vi "RT_Control_Adrian_ESP.vi"(10 "rt fifo":refnum<k33>, 11 "Parameters":T1={"N_chan"=0, "Input Rate (Hz)"=0.0, "Acq Time (s)"=0.0, "NumOfWarmupIters"=0, "Size fifo"=0, "Period NCL (ms)"=0, "Timeout fifo Read"=0, "Size Sent Array"=0, "Output offsets"=[], "Input offsets"=[0.0, 0.0, 0.0, 0.0, 0.0, 0.0, 0.0, 0.0]}) -> (0 "error out":errorcluster, 2 "Delayed Cycles":dbl)   [LabVIEW 2021]
uses:
  parametersRT.ctl
  <vilib>/DAQmx/write.llb/DAQmx Write (Analog 1D DBL NChan 1Samp).vi
  <vilib>/DAQmx/read.llb/DAQmx Read (Analog 1D DBL NChan 1Samp).vi
  <vilib>/DAQmx/write.llb/DAQmx Write (Digital Bool 1Line 1Point).vi
  <vilib>/DAQmx/create/channels.llb/DAQmx Create Channel (DO-Digital Output).vi
  <vilib>/DAQmx/configure/timing.llb/DAQmx Timing (Sample Clock).vi
  <vilib>/DAQmx/miscellaneous.llb/DAQmx Fill In Error Info.vi
  <resource>/objmgr/daqmx.rc
panel:
  out "timed out?":bool
  out "# elements":u32
  out "data":dbl[](array[numeric]) format="%0.2f"
  out "Numeric":i32
  out "output array":dbl[](array[numeric])
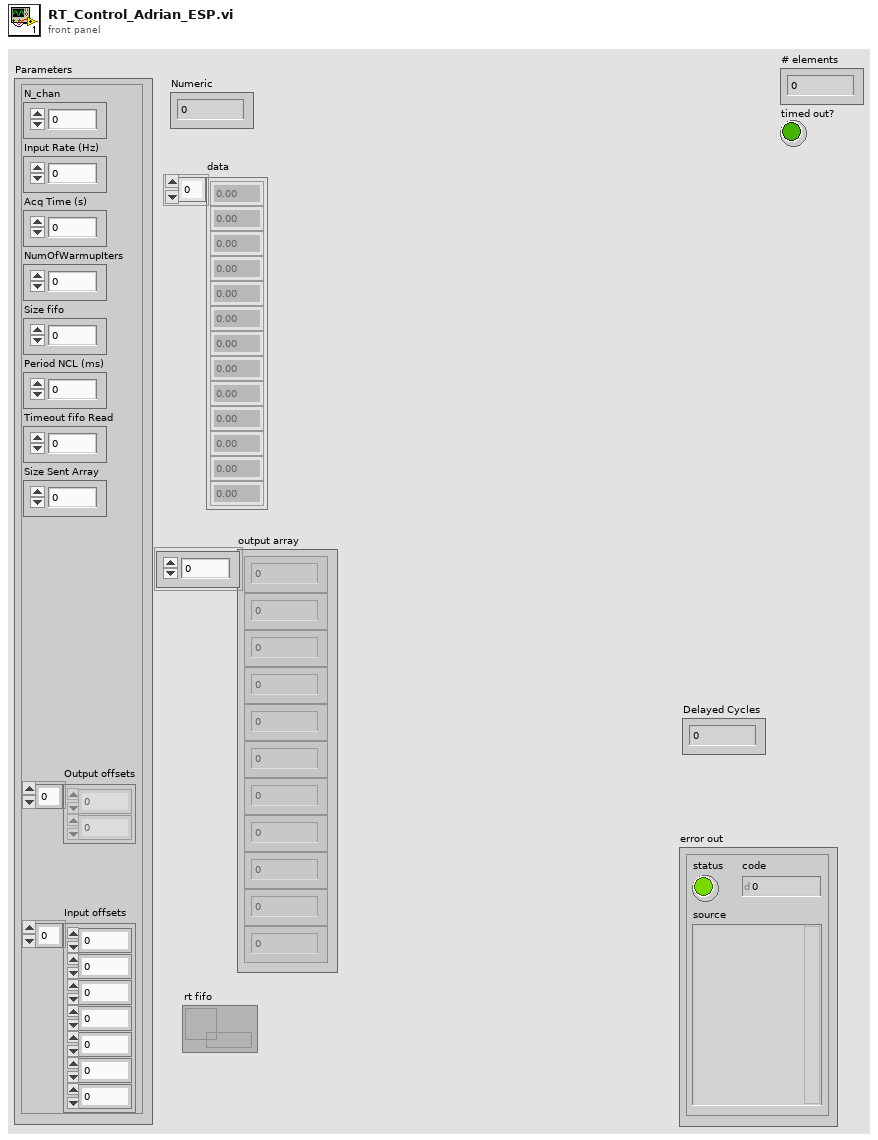
[diagram p1: front panel]
types:
  T1 = typedef "parametersRT.ctl" = cluster{"N_chan":u32, "Input Rate (Hz)":dbl, "Acq Time (s)":dbl, "NumOfWarmupIters":u32, "Size fifo":u32, "Period NCL (ms)":i64, "Timeout fifo Read":i32, "Size Sent Array":i32, "Output offsets":dbl[], "Input offsets":dbl[]}
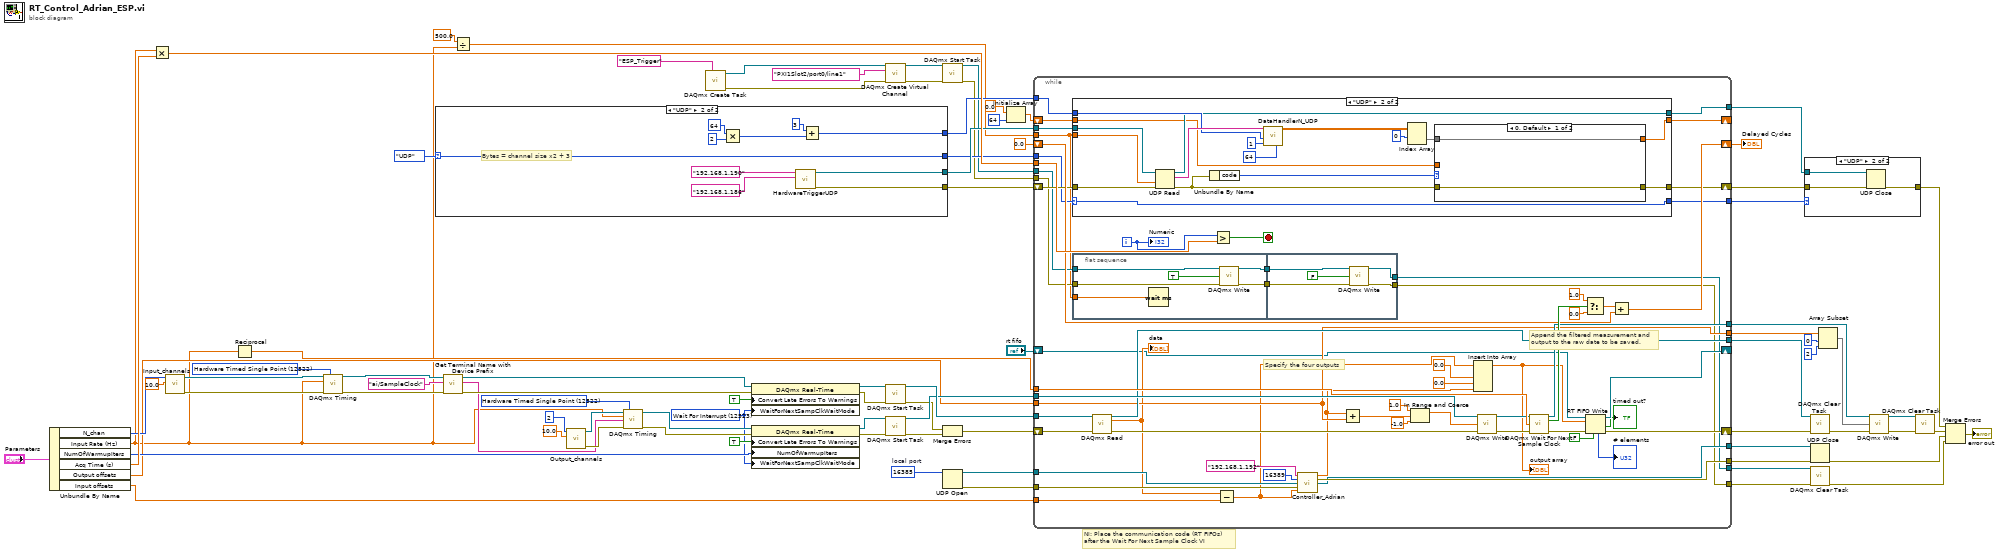
[diagram p0: block diagram]
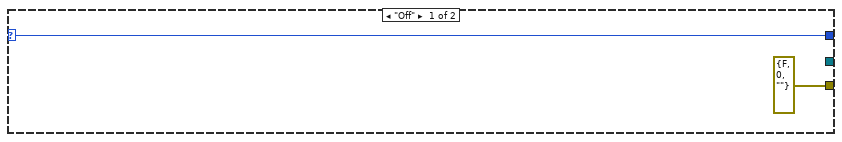
[diagram p3: hidden frame]
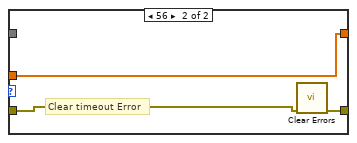
[diagram p5: hidden frame]
diagram:
  w42 = u16 16385  # local port
  w49 = 12522 items=["Finite Samples"=10178, "Continuous Samples"=10123, "Hardware Timed Single Point"=12522] ("sample mode")
  w57 = 12523 items=["Wait For Interrupt"=12523, "Poll"=12524, "Yield"=12525] ("WaitForNextSampClkWaitMode")
  w83 = 12522 items=["Finite Samples"=10178, "Continuous Samples"=10123, "Hardware Timed Single Point"=12522] ("sample mode")
  # "NI: Place the communication code (RT FIFOs) \nafter the Wait For Next Sample Clock VI"
  n1 = Unbundle By Name("Parameters") -> ("N_chan"=w68:u32, "Input Rate (Hz)"=w17:dbl, "NumOfWarmupIters"=w69:u32, "Acq Time (s)"=w76:dbl, "Output offsets"=w67:dbl[], "Input offsets"=w58:dbl[])
  n2 = Multiply(x=w17, y=w76) -> (x*y=w36:dbl)
  n3 = call "Input_channels.vi"("Range"=10.0, "nchan"=w68) -> ("error out"=w51:errorcluster, "Refnum out"=w50:refnum<k21>)  [unwired: 8 in]
  n4 = Reciprocal(x=w17) -> (1/x=w82:dbl)
  n5 = call-poly <vilib>:"DAQmx Timing.vi"("task/channels in"=w50, "sample mode"=w49, "rate"=w17, "error in"=w51) -> ("task out"=w30:refnum<k21>, "error out"=w32:errorcluster)  [unwired: 10 in]
  n6 = case shown="\"UDP\"" enum16{"Off", "UDP"}."UDP" {
    selector: enum16{"Off", "UDP"}."UDP" -> [w86 w89]
    tunnel: [_ w92] -> w23
    tunnel: [errorcluster {"status"=FALSE, "code"=0, "source"=""} ("error constant") w90] -> w25
    tunnel: [w86 w89] -> w22
    tunnel: [_ w88] -> w24
    frame "Off" {
    }
    frame "UDP" {
      # "Bytes = channel size x2 + 3"
      n7 = Multiply(x=64, y=2) -> (x*y=w95:i32)
      n8 = call "HardwareTriggerUDP.vi"("Local IP address"="192.168.1.186" ("Hardware Trigger"), "Remote IP address"="192.168.1.190" ("IP address")) -> ("error out"=w90:errorcluster, "connection ID out"=w88:refnum<k16>)  [unwired: 8 in]
      n9 = Add(x=3, y=w95) -> (x+y=w92:i32)
    }
  }
  n10 = call "Get Terminal Name with Device Prefix.vi"("error in (no error)"=w32, "Local Terminal Name"="ai/SampleClock", "task/channels in"=w30) -> ("error out"=w31:errorcluster, "Terminal Name with Device Prefix"=w28:tag, "task out"=w29:refnum<k21>)  [unwired: 6 in]
  n11 = Divide(x=500.0, y=w17) -> (x/y=w16:dbl)
  n12 = call "Output_channels.vi"("Range"=10.0 ("Maximum Value"), "nchan"=2) -> ("error out"=w73:errorcluster, "Refnum out"=w72:refnum<k21>)  [unwired: 8 in]
  n13 = call-poly <vilib>:"DAQmx Timing.vi"("task/channels in"=w72, "sample mode"=w83, "rate"=w17, "source"=w28, "error in"=w73) -> ("task out"=w81:refnum<k21>, "error out"=w80:errorcluster)  [unwired: 9 in]
  n14 = call <vilib>:"DAQmx Create Task.vi"("new task name"="ESP_Trigger") -> ("task out"=w13:refnum<k21>, "error out"=w12:errorcluster)  [unwired: 13 in]
  n15 = property class="DAQmx Real-Time"(reference=w29, error in=w31, "Convert Late Errors To Warnings"=TRUE, "WaitForNextSampClkWaitMode"=w57) -> (reference out=w46:refnum<k21>, error out=w45:errorcluster)
  n16 = property class="DAQmx Real-Time"(reference=w81, error in=w80, "Convert Late Errors To Warnings"=TRUE, "NumOfWarmupIters"=w69, "WaitForNextSampClkWaitMode"=w57) -> (reference out=w77:refnum<k21>, error out=w54:errorcluster)
  n17 = call-poly <vilib>:"DAQmx Create Virtual Channel.vi"("task in"=w13, "lines"=tag "PXI1Slot2/port0/line1", "error in"=w12) -> ("task out"=w11:refnum<k21>, "error out"=w10:errorcluster)  [unwired: 11 in]
  n18 = call <vilib>:"DAQmx Start Task.vi"("task/channels in"=w46, "error in"=w45) -> ("task out"=w75:refnum<k21>, "error out"=w44:errorcluster)  [unwired: 12 in]
  n19 = call <vilib>:"DAQmx Start Task.vi"("task/channels in"=w77, "error in"=w54) -> ("task out"=w74:refnum<k21>, "error out"=w53:errorcluster)  [unwired: 12 in]
  n20 = call <vilib>:"DAQmx Start Task.vi"("task/channels in"=w11, "error in"=w10) -> ("task out"=w8:refnum<k21>, "error out"=w9:errorcluster)  [unwired: 12 in]
  n21 = Merge Errors(w44, w53) -> (w43:errorcluster)
  n22 = UDP Open(11:w42) -> (port=w40:refnum<k16>, 0:w41:errorcluster)  [unwired: 4 in, 1 out]
  n23 = Initialize Array(0.0, 64) -> (w19:dbl[])
  n24 = while {
    shift-right: [w122] -> w52
    shift-left: w43 -> [w140]
    shift-right: [w152] -> w84
    shift-left: 0.0 ("f") -> [w127]
    tunnel: w82 -> [w150]
    tunnel: w36 -> [w148]
    tunnel: w74 -> [w146]
    tunnel: [w141] -> w78
    tunnel: w75 -> [w142]
    tunnel: [w144] -> w66
    tunnel: w67 -> [w135]
    tunnel: [w135] -> w61
    tunnel: w58 -> [w143]
    tunnel: w41 -> [w133]
    tunnel: w40 -> [w132]
    tunnel: [w131] -> w39
    tunnel: [w130] -> w38
    shift-right: [w118] -> _
    shift-left: "rt fifo" -> [w119]
    tunnel: w24 -> [w111]
    tunnel: w23 -> [w110]
    tunnel: w22 -> [w109]
    tunnel: w16 -> [w103]
    tunnel: w9 -> [w105]
    tunnel: w8 -> [w104]
    tunnel: [w102] -> w7
    tunnel: [w101] -> w6
    tunnel: [w100] -> w4
    tunnel: [w99] -> w3
    shift-right: [w98] -> _
    shift-left: w19 -> [w108]
    shift-right: [w97] -> w1
    shift-left: w25 -> [w112]
    i -> [w125]
    stop <- w149 stop-if-true
    # "Append the filtered measurement and \noutput to the raw date to be saved."
    # "Specify the four outputs"
    n25 = case shown="\"UDP\"" w109 {
      selector: w109 -> [w170 w184]
      tunnel: w110 -> [_ w186]
      tunnel: w112 -> [w169 w185]
      tunnel: [w169 w178] -> w97
      tunnel: [w170 w184] -> w99
      tunnel: [w167 w175] -> w98
      tunnel: w103 -> [_ w171]
      tunnel: w111 -> [w168 w177]
      tunnel: [w168 w176] -> w100
      tunnel: w108 -> [w167 w174]
      frame "Off", Default {
      }
      frame "UDP" {
        n26 = UDP Read(connection ID=w177, timeout ms (25000)=w171, 8:w185) -> (data out=w187:string, error out=w179:errorcluster, 3:w176:refnum<k16>)  [unwired: 1 in, 2 out]
        n27 = Unbundle By Name(w179) -> ("code"=w180:i32)
        n28 = call "DataHandlerN_UDP.vi"("Data Cycles Per Buffer"=1, "Rx Packet Byte size"=w186, "data out"=w187, "Nchan"=64) -> ("Data"=w172:sgl[][])  [unwired: 1 in, 4 out]
        n29 = Index Array(array=w172, index (row)=0 ("Data Cycles Per Buffer")) -> (element=w173:sgl[])  [unwired: 1 in]
        n30 = case shown="0, Default" w180 {
          tunnel: w179 -> [w189 w192]
          tunnel: [w189 w191] -> w178
          tunnel: w173 -> [w188 _]
          tunnel: [w188 w190] -> w175
          tunnel: w174 -> [_ w190]
          frame 0, Default {
          }
          frame 56 {
            # "Clear timeout Error"
            n31 = call <vilib>:"Clear Errors.vi"("error in (no error)"=w192) -> ("error out"=w191:errorcluster)  [unwired: 5 in, 1 out]
          }
        }
      }
    }
    n32 = flat-sequence {
      tunnel: w105 -> [w161]
      tunnel: w104 -> [w160]
      tunnel: [w159] -> w107
      tunnel: [w158] -> w106
      tunnel: w103 -> [w156]
      tunnel: [w164] -> w101
      tunnel: [w165] -> w102
      tunnel: w107 -> [w166]
      tunnel: w106 -> [w163]
      frame #0 {
        n33 = Wait (ms)(milliseconds to wait=w156) -> ()  [unwired: 1 out]
        n34 = call-poly <vilib>:"DAQmx Write.vi"("task/channels in"=w160, "data"=TRUE, "error in"=w161) -> ("task out"=w158:refnum<k21>, "error out"=w159:errorcluster)  [unwired: 10 in, 1 out]
      }
      frame #1 {
        n35 = call-poly <vilib>:"DAQmx Write.vi"("task/channels in"=w163, "data"=FALSE, "error in"=w166) -> ("task out"=w164:refnum<k21>, "error out"=w165:errorcluster)  [unwired: 10 in, 1 out]
      }
    }
    n36 = call-poly <vilib>:"DAQmx Read.vi"("task/channels in"=w142, "error in"=w140) -> ("task out"=w141:refnum<k21>, "data"=w124:dbl[], "error out"=w139:errorcluster)  [unwired: 11 in]
    "data" <- w124
    n37 = Greater?(x=w125, y=w148) -> (0:w149:bool)
    n38 = Subtract(x=w124, y=w143) -> (x-y=w126:dbl[])
    n39 = call "Controller_Adrian.vi"("name 2"="192.168.1.192", "port or service name"=u16 16389, "connection ID"=w132, "error in (no error)"=w133, "x"=w126) -> ("*(type *) &x"=w117:dbl[], "error out"=w131:errorcluster, "connection ID out"=w130:refnum<k16>)  [unwired: 8 in]
    n40 = Add(x=w117, y=w135) -> (x+y=w137:dbl[])
    n41 = In Range and Coerce(upper limit=1.0, x=w137, lower limit=-1.0) -> (coerced(x)=w134:dbl[])  [unwired: 1 out]
    n42 = Insert Into Array(array=w126, new element #1=0.0 ("new element/subarray"), new element #2=0.0 ("new element/subarray"), new element #3=w117) -> (w120:dbl[])  [unwired: 1 in]
    "output array" <- w120
    n43 = call-poly <vilib>:"DAQmx Write.vi"("task/channels in"=w146, "data"=w134, "error in"=w139) -> ("task out"=w145:refnum<k21>, "error out"=w147:errorcluster)  [unwired: 10 in, 1 out]
    n44 = call <vilib>:"DAQmx Wait For Next Sample Clock.vi"("task/channels in"=w145, "timeout (sec)"=w150, "error in"=w147) -> ("task out"=w144:refnum<k21>, "is late?"=w151:bool, "error out"=w121:errorcluster)  [unwired: 10 in]
    n45 = Select(t=1.0, s=w151, f=0.0) -> (s? t:f=w153:dbl)
    n46 = RT FIFO Write(0:w119, 1:w120, 3:w121, 5:FALSE ("overwrite on timeout (T)")) -> (7:→"# elements":u32, 8:w118:refnum<k33>, 10:→"timed out?":bool, 11:w122:errorcluster)  [unwired: 1 in]
    n47 = Add(x=w153, y=w127) -> (x+y=w152:dbl)
    "Numeric" <- w125
  }
  "Delayed Cycles" <- w84
  n48 = case shown="\"UDP\"" w3 {
    tunnel: w1 -> [w193 w196]
    tunnel: [w193 w195] -> w2
    tunnel: w4 -> [_ w194]
    frame "Off", Default {
    }
    frame "UDP" {
      n49 = UDP Close(connection ID=w194, 8:w196) -> (error out=w195:errorcluster)  [unwired: 1 out]
    }
  }
  n50 = call <vilib>:"DAQmx Clear Task.vi"("task in"=w78, "error in"=w52) -> ("error out"=w64:errorcluster)  [unwired: 13 in]
  n51 = call <vilib>:"DAQmx Clear Task.vi"("task in"=w6, "error in"=w7) -> ("error out"=w5:errorcluster)  [unwired: 13 in]
  n52 = UDP Close(connection ID=w38, 8:w39) -> (error out=w37:errorcluster)  [unwired: 1 out]
  n53 = Array Subset(array=w61, index=0, length=2) -> (w62:dbl[])
  n54 = call-poly <vilib>:"DAQmx Write.vi"("task/channels in"=w66, "data"=w62, "error in"=w64) -> ("task out"=w65:refnum<k21>, "error out"=w63:errorcluster)  [unwired: 10 in, 1 out]
  n55 = call <vilib>:"DAQmx Clear Task.vi"("task in"=w65, "error in"=w63) -> ("error out"=w56:errorcluster)  [unwired: 13 in]
  n56 = Merge Errors(w2, w56, w37, w5) -> (→"error out":errorcluster)
